vi "Generate 2D scan Waveform.vi"(8 "error in (no error)":errorcluster, 11 "System Parameters [In]":T1={"Optical /HW Parameters"={"Focal Length [mm]"=0.0, "Scan Lens EFL[mm]"=0.0, "Tube Lens EFL[mm]"=0.0, "Galvo V Range (+/-)"=0.0, "Galvo Max Half Angle [Deg]"=0.0, "Max Galvo Range[%]"=0.0}, "Vibratome"={"Z Bottom [mm]"=0.0, "Pre Cut Dwell [s]"=0.0, "Blade Frequency [RPM]"=0, "Slice Speed [mm/s]"=0.0, "Post Cut Dwell [s]"=0.0, "Ramp Time [s]"=0.0, "Start X [mm]"=0.0, "Start Y [mm]"=0.0, "Slice Length [mm]"=0.0, "Slice Axis"=enum."Y Axis", "Controller VISA Ref"="COM4"}, "Table Stages"={"X Stage"={"Position"=0.0, "Is.Enabled?"=FALSE, "Is.Connected?"=FALSE, "Device SN"="45876539", "AccelerationMaximum"=0.0, "VelocityMaximum"=0.0, "Acceleration"=0.0, "Velocity"=0.0, "waitTimeout (ms)"=0, "Model"=enum."None", "Is.Homed?"=FALSE}, "Y Stage"={"Position"=0.0, "Is.Enabled?"=FALSE, "Is.Connected?"=FALSE, "Device SN"="45876539", "AccelerationMaximum"=0.0, "VelocityMaximum"=0.0, "Acceleration"=0.0, "Velocity"=0.0, "waitTimeout (ms)"=0, "Model"=enum."None", "Is.Homed?"=FALSE}, "Z Stage"={"Position"=0.0, "Is.Enabled?"=FALSE, "Is.Connected?"=FALSE, "Device SN"="45876539", "AccelerationMaximum"=0.0, "VelocityMaximum"=0.0, "Acceleration"=0.0, "Velocity"=0.0, "waitTimeout (ms)"=0, "Model"=enum."None", "Is.Homed?"=FALSE}}, "Imaging Parameter"={"Raster Scan Direction"=enum."Uni Directional", "Pixel Dwell Time [Clock Cycles]"=0, "Flyback Time [Clock Cycles]"=0, "XY Center [um]"={"X"=1.0, "Y"=1.0}, "Pixel Step Size [um]"=1.0, "XY Image Resolution"=enum."256 x 256", "Custom"=FALSE, "Custom Size"={"X"=1, "Y"=1}, "Line Averages"=1}} {"Imaging Parameter"."Line Averages" min=1 max=30 step=1; "Imaging Parameter"."Flyback Time [Clock Cycles]" max=10 step=1; "Imaging Parameter"."Pixel Step Size [um]" min=0.0 max=10.0 step=0.01; "Imaging Parameter"."Custom Size"."Y" min=1 max=30 step=1; "Imaging Parameter"."Custom Size"."X" min=1 max=30 step=1; "Imaging Parameter"."XY Center [um]"."Y" min=1.0 max=30.0 step=1.0; "Imaging Parameter"."XY Center [um]"."X" min=1.0 max=30.0 step=1.0; "Imaging Parameter"."Pixel Dwell Time [Clock Cycles]" max=1000 step=1}) -> (0 "error out":errorcluster, 2 "Digital Line Acq":bool[](array[boolean]), 3 "Array 3":dbl[][](array[numeric]))   [LabVIEW 2018]
uses:
  Controls/System Parameters.ctl
  Hardware/Table Stage/Controls/Translation Stage Cluster.ctl
  Controls/Translation Stage Types.ctl
  Controls/Scan Direction.ctl
panel:
  out "dt":dbl
  # "X"
  # "X"
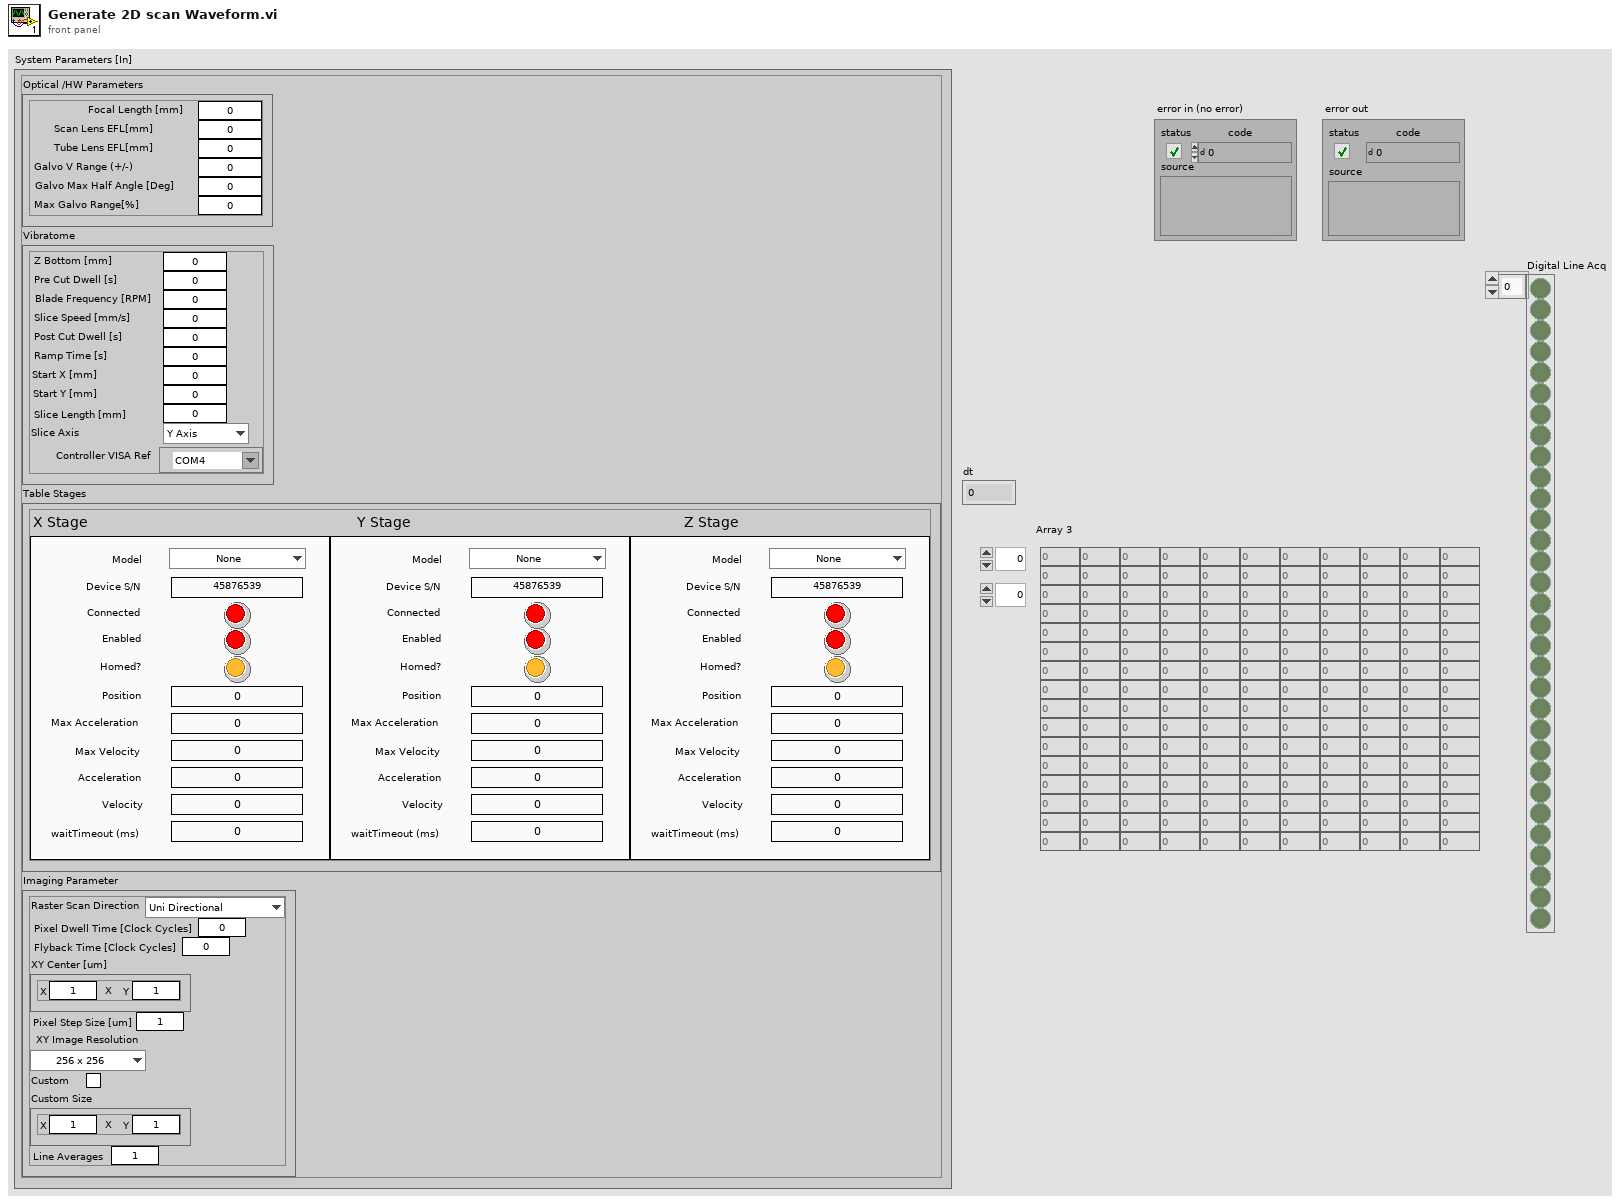
[diagram p1: front panel]
types:
  T1 = typedef "System Parameters.ctl" = cluster{"Optical /HW Parameters":cluster{"Focal Length [mm]":dbl, "Scan Lens EFL[mm]":dbl, "Tube Lens EFL[mm]":dbl, "Galvo V Range (+/-)":dbl, "Galvo Max Half Angle [Deg]":dbl, "Max Galvo Range[%]":dbl}, "Vibratome":cluster{"Z Bottom [mm]":dbl, "Pre Cut Dwell [s]":dbl, "Blade Frequency [RPM]":u16, "Slice Speed [mm/s]":dbl, "Post Cut Dwell [s]":dbl, "Ramp Time [s]":dbl, "Start X [mm]":dbl, "Start Y [mm]":dbl, "Slice Length [mm]":dbl, "Slice Axis":enum16{"X Axis", "Y Axis", "Z Axis"}, "Controller VISA Ref":refnum<visa-resource-name>}, "Table Stages":cluster{"X Stage":T2, "Y Stage":T2, "Z Stage":T2}, "Imaging Parameter":cluster{"Raster Scan Direction":T4, "Pixel Dwell Time [Clock Cycles]":u16, "Flyback Time [Clock Cycles]":u16, "XY Center [um]":cluster{"X":dbl, "Y":dbl}, "Pixel Step Size [um]":dbl, "XY Image Resolution":enum16{"32 x 32", "64 x 64", "128 x 128", "256 x 256", "512 x 512", "1024 x 1024", "2048 x 2048"}, "Custom":bool, "Custom Size":cluster{"X":u16, "Y":u16}, "Line Averages":u8}}
  T2 = typedef "Translation Stage Cluster.ctl" = cluster{"Position":dbl, "Is.Enabled?":bool, "Is.Connected?":bool, "Device SN":string, "AccelerationMaximum":dbl, "VelocityMaximum":dbl, "Acceleration":dbl, "Velocity":dbl, "waitTimeout (ms)":i32, "Model":T3, "Is.Homed?":bool}
  T3 = typedef "Translation Stage Types.ctl" = enum16{"None", "Thorlabs LTS", "Thorlabs MLJ"}
  T4 = typedef "Scan Direction.ctl" = enum16{"Uni Directional", "Bi Directional", "None"}
  T5 = cluster{"Raster Scan Direction":T4, "Pixel Dwell Time [Clock Cycles]":u16, "Flyback Time [Clock Cycles]":u16, "XY Center [um]":cluster{"X":dbl, "Y":dbl}, "Pixel Step Size [um]":dbl, "XY Image Resolution":enum16{"32 x 32", "64 x 64", "128 x 128", "256 x 256", "512 x 512", "1024 x 1024", "2048 x 2048"}, "Custom":bool, "Custom Size":cluster{"X":u16, "Y":u16}, "Line Averages":u8}
  T6 = enum16{"32 x 32", "64 x 64", "128 x 128", "256 x 256", "512 x 512", "1024 x 1024", "2048 x 2048"}
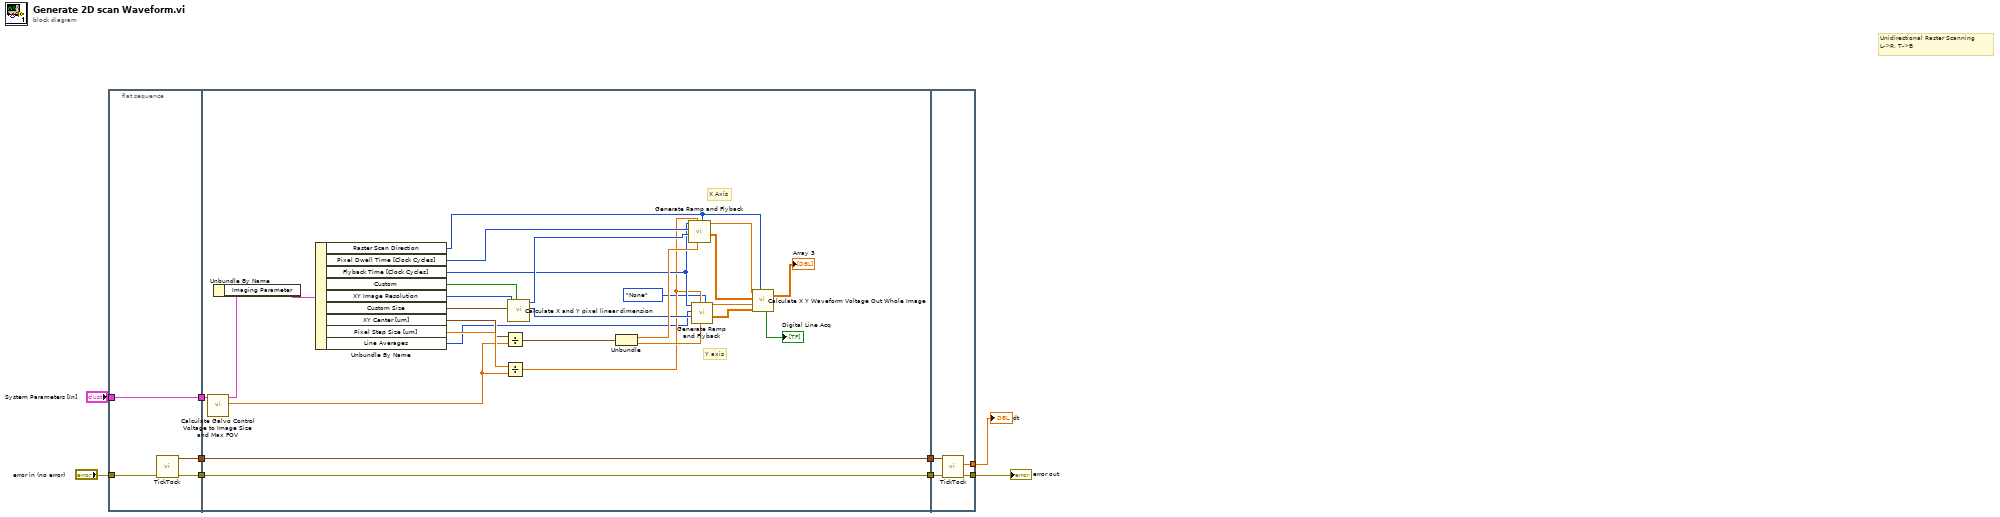
[diagram p0: block diagram]
diagram:
  # "Unidirectional Raster Scanning\nL->R, T->B"
  n1 = flat-sequence {
    tunnel: "System Parameters [In]" -> [w13]
    tunnel: [w13] -> w8
    tunnel: [w12] -> w6
    tunnel: [w11] -> w4
    tunnel: "error in (no error)" -> [w10]
    tunnel: w8 -> [w40]
    tunnel: [w17] -> w7
    tunnel: w6 -> [w17]
    tunnel: [w16] -> w5
    tunnel: w4 -> [w16]
    tunnel: w7 -> [w45]
    tunnel: w5 -> [w44]
    tunnel: [w43] -> w3
    tunnel: [w42] -> w1
    frame #0 {
      n2 = call "TickTock.vi"("Error In"=w10) -> ("Error Out"=w12:errorcluster, "Current Time (Out)"=w11:timestamp)  [unwired: 8 in, 1 out]
    }
    frame #1 {
      # "X Axis"
      # "Y axis"
      n3 = call "Calculate Galvo Control Voltage to Image Size and Max FOV.vi"("System Parameters [In]"=w40) -> ("Galvo [um/V]"=w32:dbl, "System Parameters [Out]"=w39:T1)  [unwired: 7 in, 2 out]
      n4 = Unbundle By Name(w39) -> ("Imaging Parameter"=w41:T5)
      n5 = Unbundle By Name(w41) -> ("Raster Scan Direction"=w18:T4, "Pixel Dwell Time [Clock Cycles]"=w30:u16, "Flyback Time [Clock Cycles]"=w28:u16, "Custom"=w35:bool, "XY Image Resolution"=w38:T6, "Custom Size"=w37:cluster{"X":u16, "Y":u16}, "XY Center [um]"=w33:cluster{"X":dbl, "Y":dbl}, "Pixel Step Size [um]"=w34:dbl, "Line Averages"=w24:u8)
      n6 = Divide(x=w33, y=w32) -> (x/y=w36:cluster{"X":dbl, "Y":dbl})
      n7 = Divide(x=w34, y=w32) -> (x/y=w25:dbl)
      n8 = call "Calculate X and Y pixel linear dimension.vi"("Imaging Parameter.Custom"=w35, "Custom Size"=w37, "XY Image Resolution"=w38) -> ("Y Px Dim (HFOV)"=w27:u16, "X Px Dim (HFOV)"=w29:u16)  [unwired: 5 in, 2 out]
      n9 = Unbundle(w36) -> ("X"=w31:dbl, "Y"=w26:dbl)
      n10 = call "Generate Ramp and Flyback.vi"("Raster Scan Direction"=w18, "FOV Center (V)"=w31, "Galvo Step Size Voltages (px/V)"=w25, "Px Dim (HFOV)"=w29, "Pixel Dwell Time [Clock Cycles]"=w30, "Flyback Time [Clock Cycles]"=w28) -> ("Flyback"=w21:dbl[][], "Waveform Graph"=w19:dbl[])  [unwired: 3 in, 1 out]
      n11 = call "Generate Ramp and Flyback.vi"("Raster Scan Direction"=Scan_Direction."None", "FOV Center (V)"=w26, "Galvo Step Size Voltages (px/V)"=w25, "Px Dim (HFOV)"=w27, "Pixel Dwell Time [Clock Cycles]"=w24, "Flyback Time [Clock Cycles]"=w28) -> ("Flyback"=w22:dbl[][], "Waveform Graph"=w20:dbl[])  [unwired: 3 in, 1 out]
      n12 = call "Calculate X Y Waveform Voltage Out Whole Image.vi"("Raster Scan Direction"=w18, "Y Flyback"=w22, "Y Waveform"=w20, "X Flyback"=w21, "X Waveform"=w19) -> ("Digital Line Acq"=→"Digital Line Acq":bool[], "XY Waveform Out"=→"Array 3":dbl[][])  [unwired: 3 in, 2 out]
    }
    frame #2 {
      n13 = call "TickTock.vi"("Error In"=w45, "Current Time (In)"=w44) -> ("Error Out"=w42:errorcluster, "dt"=w43:dbl)  [unwired: 7 in, 1 out]
    }
  }
  "dt" <- w3
  "error out" <- w1
